vi "Get laser device handle.vi"(1 "Selected laser":T1 items=["Green Laser", "Blue Laser"]) -> (0 "Device handle":u64)   [LabVIEW 2018]
uses:
  Laser enum.ctl
  Coherent global.vi
panel:
  # "PN 04/11/2014\n      08/04/2019"
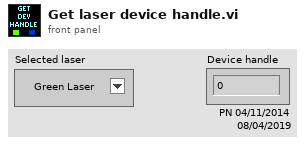
[diagram p1: front panel]
types:
  T1 = typedef "Laser enum.ctl" = u8
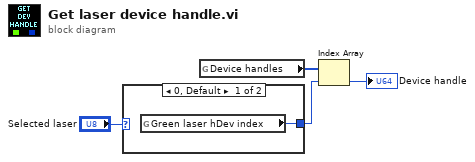
[diagram p0: block diagram]
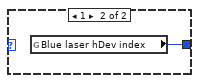
[diagram p2: hidden frame]
diagram:
  n1 = case shown="0, Default" "Selected laser" {
    tunnel: [w5 w6] -> w2
    frame 0, Default {
      n2 = global read "Coherent global.vi" "Green laser hDev index"() -> (w5:i32)
    }
    frame 1 {
      n3 = global read "Coherent global.vi" "Blue laser hDev index"() -> (w6:i32)
    }
  }
  n4 = global read "Coherent global.vi" "Device handles"() -> (w3:u64[])
  n5 = Index Array(array=w3, index=w2) -> (element=→"Device handle":u64)
